vi "Main Pipeline.vi"() -> ()   [LabVIEW 2014]
uses:
  <vilib>/sound2/lvsound2.llb/Sound File Position.ctl
  <vilib>/addons/_NISVFA/_Baseband FFT/SVFA FFT Spectrum (Mag-Phase) (N Ch).vi
  <vilib>/addons/Digital Filter Design/Process.llb/DFD Filtering (Array).vi
  <vilib>/measure/maspectr.llb/FFT Spectrum (Mag-Phase) for 1 Chan.vi
  <vilib>/addons/Digital Filter Design/NI_DigFilterLicensed.lvlib
  <vilib>/measure/NI_MAPro.lvlib
panel:
  out "normalized fft":picture
  out "max value 2":dbl
  out "max value":dbl
  out "error out":errorcluster
  out "postfilter fft":picture
  out "prefilter fft":picture
  in  "path":path
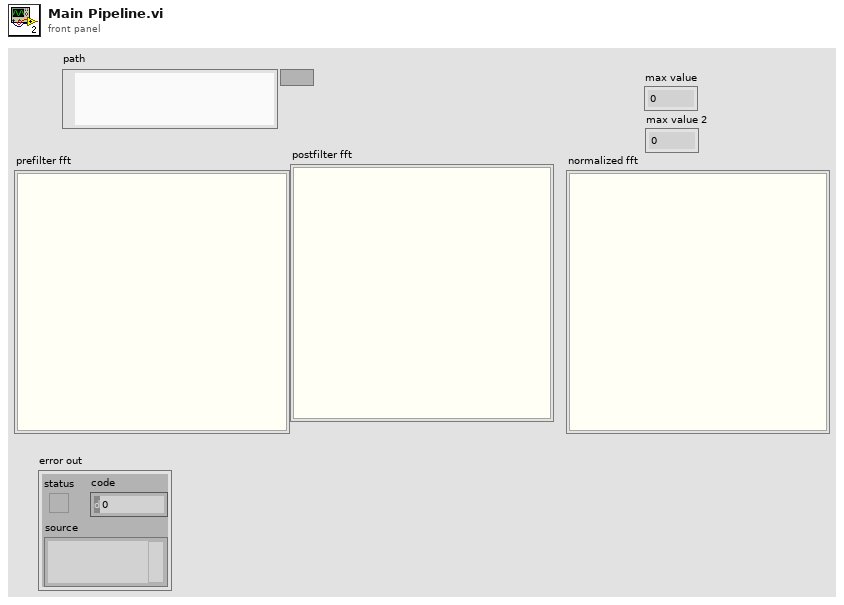
[diagram p1: front panel]
types:
  T1 = cluster{"dB On (T)":bool, "unwrap phase (F)":bool, "convert to degree (T)":bool}
  T2 = typedef "Sound File Position.ctl" = u16
  T3 = typedef "NI_DigFilterLicensed.lvlib/DFD Filter Obj.ctl" = cluster{"mSRate_Fs":dbl, "mSRate_Version":string, "mSRate_Comments":string, "mSRate_OrgCoef":T4, "mSRate_CurCoef":T4, "mSRate_Quantized?":bool, "mSRate_QCoef":T4, "mSRate_QSettings":T6[], "mSRate_Order":i32, "mSRate_Scaling":cluster{"mSRate_ScaleByPowerOf2?":bool, "mSRate_ScaleType":T8}}
  T4 = typedef "NI_DigFilterLicensed.lvlib/DFD Filter Coef.ctl" = cluster{"type":T5, "gain":dbl, "coef a (k)":dbl[], "coef b (v)":dbl[]}
  T5 = typedef "NI_DigFilterLicensed.lvlib/DFD Filter Structure Type Selector.ctl" = enum16{"Undefined", "FIR Direct Form", "FIR Direct Form Transposed", "FIR Symmetric", "FIR Antisymmetric", "IIR Direct Form I", "IIR Direct Form I Transposed", "IIR Direct Form II", "IIR Direct Form II Transposed", "IIR Cascaded Second Order Sections Form I", "IIR Cascaded Second Order Sections Form I Transposed", "IIR Cascaded Second Order Sections Form II", "IIR Cascaded Second Order Sections Form II Transposed", "Lattice Allpass (basic sections)", "Lattice Allpass (one multiplier sections)", "Lattice Allpass (normalized sections)", "Lattice AR (basic sections)", "Lattice AR (one multiplier sections)", "Lattice AR (normalized sections)", "Lattice MA (minimum phase)", "Lattice MA (maximum phase)", "Lattice ARMA (basic sections)", "Lattice ARMA (one multiplier sections)", "Lattice ARMA (normalized sections)"}
  T6 = typedef "NI_DigFilterLicensed.lvlib/dfd_Internal Quantization Settings.ctl" = cluster{"source":T7, "wl":i16, "iwl":i16, "overflow mode":enum16{"Saturation", "Wrap"}, "rounding mode":enum16{"Nearest", "Truncation"}, "signed?":bool}
  T7 = typedef "NI_DigFilterLicensed.lvlib/dfd_Internal Quantization Srcs.ctl" = u16
  T8 = typedef "NI_DigFilterLicensed.lvlib/DFD Coef Norm Type.ctl" = enum16{"No Norm", "Time Domain 1-Norm", "Time Domain 2-Norm", "Time Domain Inf-Norm"}
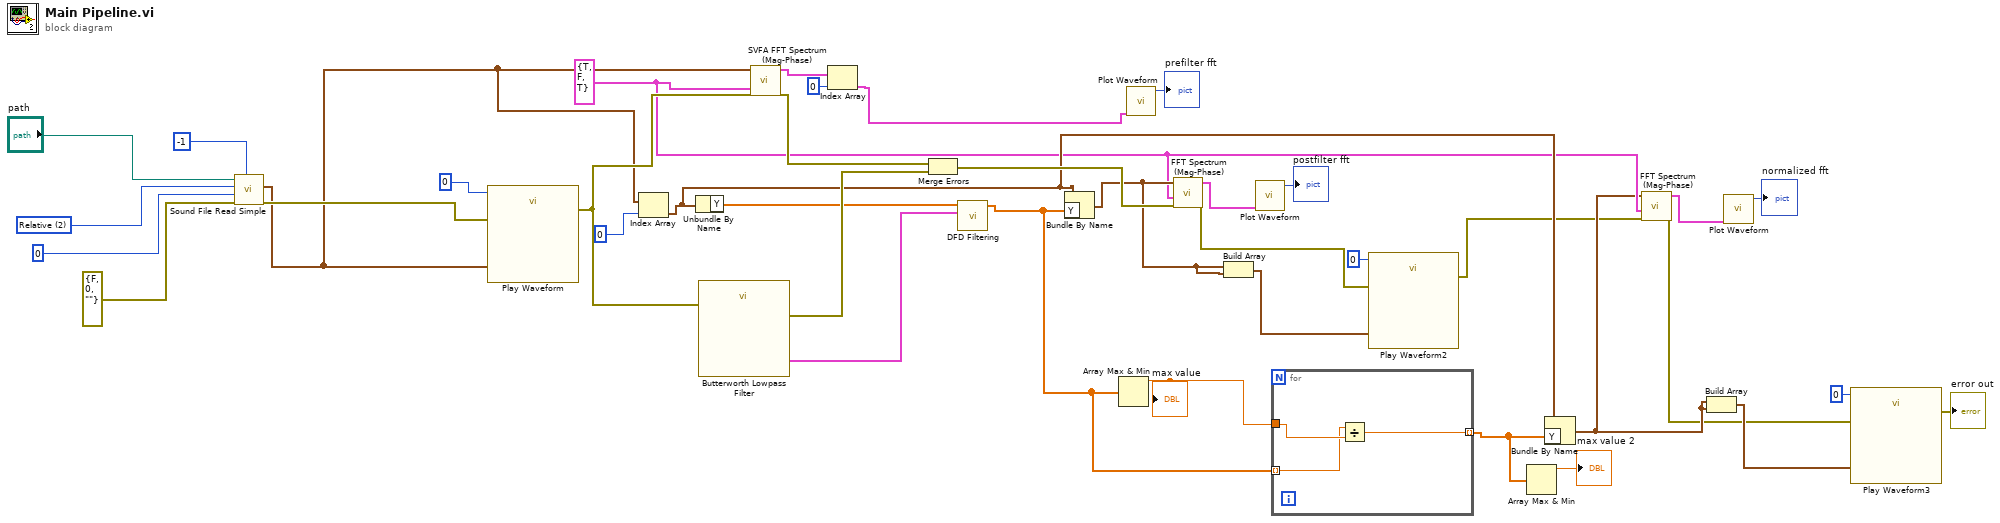
[diagram p0: block diagram]
diagram:
  w4 = T1 {"dB On (T)"=TRUE, "unwrap phase (F)"=FALSE, "convert to degree (T)"=TRUE} ("view")
  w38 = T2 2 items=["Absolute"=0, "Relative"=2] ("position mode")
  n1 = call <vilib>:"Sound File Read Simple.vi"("number of samples/ch (-1: all)"=-1, "error in (no error)"=errorcluster {"status"=FALSE, "code"=0, "source"=""}, "position offset"=0, "position mode"=w38, "path"="path") -> ("error out"=w33:errorcluster, "data"=w23:waveform(dbl)[])  [unwired: 3 in, 2 out]
  n2 = call "Play Waveform"("Device"=u32 0, "Data"=w23, "error in"=w33) -> ("error out"=w28:errorcluster)  [unwired: 16 in]
  n3 = Index Array(array=w23, index=0) -> (element=w13:waveform(dbl))
  n4 = Unbundle By Name(w13) -> ("Y"=w22:dbl[])
  n5 = call "Butterworth Lowpass Filter"("error in (no error)"=w28) -> ("error out"=w27:errorcluster, "filter out"=w25:T3)  [unwired: 9 in]
  n6 = call-poly <vilib>:"SVFA FFT Spectrum (Mag-Phase).vi"("scaled signals [EU]"=w23, "view"=w4, "error in (no error)"=w28) -> ("magnitudes [dB EU]"=w32:cluster{"f0":dbl, "df":dbl, "magnitude":dbl[]}[], "error out"=w26:errorcluster)  [unwired: 9 in, 6 out]
  n7 = Index Array(array=w32, index=0) -> (element=w30:cluster{"f0":dbl, "df":dbl, "magnitude":dbl[]})
  n8 = Merge Errors(w26, w27) -> (w21:errorcluster)
  n9 = call-poly <vilib>:"DFD Filtering.vi"("filter"=w25, "signal in"=w22) -> ("signal out"=w9:dbl[])  [unwired: 8 in, 1 out]
  n10 = Bundle By Name(cluster=w13, "Y"=w9) -> (w18:waveform(dbl))
  n11 = Array Max & Min(array=w9) -> (max value=w14:dbl)  [unwired: 3 out]
  "max value" <- w14
  n12 = call <vilib>:"Plot Waveform.vi"("waveform data"=w30) -> ("new picture"=→"prefilter fft":picture)  [unwired: 10 in]
  n13 = call-poly <vilib>:"FFT Spectrum (Mag-Phase).vi"("error in (no error)"=w21, "view"=w4, "time signal"=w18) -> ("error out"=w15:errorcluster, "magnitude"=w19:cluster{"f0":dbl, "df":dbl, "magnitude":dbl[]})  [unwired: 4 in, 3 out]
  n14 = Build Array(w18, w18) -> (w16:waveform(dbl)[])
  n15 = call <vilib>:"Plot Waveform.vi"("waveform data"=w19) -> ("new picture"=→"postfilter fft":picture)  [unwired: 10 in]
  n16 = for {
    tunnel: w9 -> [w41] mode=indexing
    tunnel: w14 -> [w42]
    tunnel: [w40] -> w8 mode=indexing
    n17 = Divide(x=w41, y=w42) -> (x/y=w40:dbl)
  }
  n18 = call "Play Waveform2"("Device"=u32 0, "Data"=w16, "error in"=w15) -> ("error out"=w2:errorcluster)  [unwired: 16 in]
  n19 = Array Max & Min(array=w8) -> (max value=→"max value 2":dbl)  [unwired: 3 out]
  n20 = Bundle By Name(cluster=w13, "Y"=w8) -> (w3:waveform(dbl))
  n21 = call-poly <vilib>:"FFT Spectrum (Mag-Phase).vi"("error in (no error)"=w2, "view"=w4, "time signal"=w3) -> ("error out"=w1:errorcluster, "magnitude"=w5:cluster{"f0":dbl, "df":dbl, "magnitude":dbl[]})  [unwired: 4 in, 3 out]
  n22 = Build Array(w3, w3) -> (w11:waveform(dbl)[])
  n23 = call <vilib>:"Plot Waveform.vi"("waveform data"=w5) -> ("new picture"=→"normalized fft":picture)  [unwired: 10 in]
  n24 = call "Play Waveform3"("Device"=u32 0, "Data"=w11, "error in"=w1) -> ("error out"=→"error out":errorcluster)  [unwired: 16 in]
